vi "PIDcontro2DCmotorUsingMyRio.vi"() -> ()   [LabVIEW 2017]
uses:
  <vilib>/myRIO/Common/Instrument Driver Framework/myRIO v1.0/Encoder/typedefs/Encoder Count Direction Enum.ctl
  <vilib>/myRIO/Common/Instrument Driver Framework/myRIO v1.0/Encoder/typedefs/Encoder Signal Mode.ctl
  <vilib>/myRIO/Instrument Drivers/Onboard IO/Encoder/typedefs/Encoder Reference.ctl
  <vilib>/myRIO/Common/Instrument Driver Framework/Utilities/typedefs/myRIO Generic Hardware Reference.ctl
  <vilib>/myRIO/Common/Instrument Driver Framework/Utilities/typedefs/Hardware Version Enum.ctl
  <vilib>/myRIO/Common/Instrument Driver Framework/Utilities/typedefs/myRIO v1.0 Reference.ctl
  <vilib>/myRIO/Common/Instrument Driver Framework/Utilities/typedefs/Generic FPGA Reference.ctl
  <vilib>/myRIO/Common/Instrument Driver Framework/myRIO v1.0/Encoder/typedefs/Encoder Channels Enum.ctl
  <vilib>/myRIO/Common/Instrument Driver Framework/myRIO v1.0/Encoder/typedefs/Encoder Configuration v1.0.ctl
  <vilib>/userdefined/High Color/nirio_resource_hc.ctl
  <vilib>/myRIO/Instrument Drivers/Onboard IO/PWM/typedefs/PWM Reference.ctl
  <vilib>/myRIO/Common/Instrument Driver Framework/myRIO v1.0/PWM/typedefs/PWM Channels Enum.ctl
  <vilib>/myRIO/Instrument Drivers/Onboard IO/PWM/typedefs/PWM Configuration.ctl
  <vilib>/myRIO/Instrument Drivers/Onboard IO/DIO/typedefs/DIO Reference.ctl
  <vilib>/myRIO/Common/Instrument Driver Framework/myRIO v1.0/DIO/typedefs/DIO Channels List.ctl
  <vilib>/myRIO/Common/Instrument Driver Framework/myRIO v1.0/DIO/typedefs/DIO Channels Enum.ctl
  <vilib>/myRIO/Common/Instrument Driver Framework/Utilities/vis/Is FPGA Ref Available.vi
  <vilib>/myRIO/Common/Instrument Driver Framework/myRIO v1.0/Encoder/vis/myRIO v1.1 Open Encoder.vi
  <vilib>/myRIO/Instrument Drivers/Onboard IO/Encoder/vis/Read.vi
  <vilib>/myRIO/Common/Instrument Driver Framework/myRIO v1.0/PWM/vis/myRIO v1.1 Open PWM.vi
  <vilib>/myRIO/Instrument Drivers/Onboard IO/PWM/vis/Set Duty Cycle and Frequency.vi
  <vilib>/myRIO/Common/Instrument Driver Framework/myRIO v1.0/DIO/vis/myRIO v1.1 Open DIO.vi
  <vilib>/myRIO/Instrument Drivers/Onboard IO/DIO/vis/Write.vi
  <vilib>/myRIO/Common/Instrument Driver Framework/Utilities/vis/Validate Channels.vi
  <vilib>/myRIO/Common/Instrument Driver Framework/myRIO v1.0/Encoder/vis/myRIO v1.0 Reserve Encoder.vi
  <vilib>/myRIO/Common/Instrument Driver Framework/myRIO v1.0/PWM/vis/myRIO v1.0 Reserve PWM.vi
  <vilib>/myRIO/Common/Instrument Driver Framework/myRIO v1.0/DIO/vis/myRIO v1.0 Reserve DIO.vi
  <vilib>/myRIO/Common/Instrument Driver Framework/myRIO v1.0/UART/vis/myRIO v1.0 Close UART.vi
  <vilib>/myRIO/Common/Instrument Driver Framework/myRIO v1.0/Encoder/vis/myRIO v1.0 Build MUX Configuration Encoder.vi
  <vilib>/myRIO/Common/Instrument Driver Framework/myRIO v1.0/Resource Manager/vis/myRIO v1.0 Reserve Channel List.vi
  <vilib>/myRIO/Common/Instrument Driver Framework/myRIO v1.0/PWM/vis/myRIO v1.0 Build MUX Configuration PWM.vi
  <vilib>/myRIO/Common/Instrument Driver Framework/myRIO v1.0/DIO/vis/myRIO v1.0 Build MUX Configuration DIO.vi
  <vilib>/myRIO/Common/Instrument Driver Framework/myRIO v1.0/Resource Manager/vis/myRIO v1.0 Create Configuration List.vi
  <vilib>/myRIO/Common/Instrument Driver Framework/myRIO v1.0/Resource Manager/vis/myRIO v1.0 Reserve Channel.vi
  <vilib>/myRIO/Common/Instrument Driver Framework/myRIO v1.0/Resource Manager/vis/myRIO v1.0 Unreserve Channel.vi
  <vilib>/myRIO/Common/Instrument Driver Framework/myRIO v1.0/Resource Manager/vis/myRIO v1.0 Build Mutex Name.vi
  <vilib>/myRIO/Instrument Drivers/Onboard IO/Encoder/vis/Smart Open.vi
  <vilib>/Utility/error.llb/Error Cluster From Error Code.vi
  <vilib>/myRIO/Common/Instrument Driver Framework/myRIO v1.0/Encoder/vis/myRIO v1.0 Read Encoder.vi
  <vilib>/Utility/VariantDataType/GetNumericInfo.vi
  <vilib>/myRIO/Common/Instrument Driver Framework/myRIO v1.0/myRIO v1.1 Open.vi
  <vilib>/myRIO/Common/Instrument Driver Framework/Utilities/vis/IO Manager.vi
  <vilib>/myRIO/Common/Instrument Driver Framework/Utilities/vis/Configuration Manager.vi
  <vilib>/myRIO/Common/Instrument Driver Framework/myRIO v1.0/Resource Manager/vis/myRIO v1.0 Configure IO.vi
  <vilib>/myRIO/Common/Instrument Driver Framework/myRIO v1.0/myRIO v1.0 Close.vi
  <vilib>/myRIO/Common/Instrument Driver Framework/myRIO v1.0/Encoder/vis/myRIO v1.0 Configure Encoder.vi
  <vilib>/addons/control/pid/pid.llb/PID (DBL).vi
  <vilib>/myRIO/Common/Instrument Driver Framework/myRIO v1.0/PWM/vis/myRIO v1.0 Write PWM.vi
  <vilib>/myRIO/Common/Instrument Driver Framework/myRIO v1.0/DIO/vis/myRIO v1.0 Write DIO.vi
  <vilib>/myRIO/Instrument Drivers/Onboard IO/PWM/vis/Smart Open.vi
  <vilib>/myRIO/Instrument Drivers/Onboard IO/DIO/vis/Smart Open.vi
  <vilib>/myRIO/Common/Instrument Driver Framework/Utilities/vis/FPGA Ref Manager.vi
  <vilib>/myRIO/Common/Instrument Driver Framework/myRIO v1.0/myRIO v1.0 Reset FPGA.vi
  <vilib>/myRIO/Common/Instrument Driver Framework/myRIO v1.0/IRQ/vis/myRIO v1.0 IRQ Info FGV.vi
  <vilib>/myRIO/Common/Instrument Driver Framework/myRIO v1.0/IRQ/vis/myRIO v1.0 Timer IRQ Info FGV.vi
  <vilib>/myRIO/Common/Instrument Driver Framework/myRIO v1.0/IRQ/vis/myRIO v1.0 ISR Agent.vi
  <vilib>/myRIO/Express VI/Onboard IO/Encoder/Encoder Express VI.xnode
  <vilib>/myRIO/Instrument Drivers/Onboard IO/Encoder/vis/myRIO Encoder Open.xnode
  <vilib>/myRIO/Express VI/Onboard IO/PWM/PWM Express VI.xnode
  <vilib>/myRIO/Instrument Drivers/Onboard IO/PWM/vis/myRIO PWM Open.xnode
  <vilib>/myRIO/Express VI/Onboard IO/DO/DO Express VI.xnode
  <vilib>/myRIO/Instrument Drivers/Onboard IO/DIO/vis/myRIO DIO Open.xnode
  <vilib>/myRIO/Instrument Drivers/Utilities/Utilities.lvlib
  <vilib>/addons/control/pid/NI_PID_pid.lvlib
  <vilib>/myRIO/Instrument Drivers/Onboard IO/DIO/DIO.lvlib
  <vilib>/myRIO/Instrument Drivers/Onboard IO/PWM/PWM.lvlib
  <vilib>/myRIO/Instrument Drivers/Onboard IO/Encoder/Encoder.lvlib
panel:
  in  "Enable 2":bool
  out "Direction 2":bool
  out "Counter Value 2":i32
  out "Counter Direction 2":T1
  in  "Reset Counter 2":bool
  out "PPS 2":dbl
  out "RPM 2":dbl
  out "RPS 2":dbl
  out "Motor Response-SetSpeed & ActualSpeed RightM":cluster{"Speed SetPoint":dbl, dbl}(graph)
  out "Motor Right Speed RPM RPM 2":dbl(knob) caption="Gauge" scale=0.0..150.0
  out "Motor Left Speed RPM":dbl(knob) caption="Gauge" scale=0.0..150.0
  out "Motor Response-SetSpeed & ActualSpeed LeftM":cluster{"Speed SetPoint":dbl, dbl}(graph)
  out "RPS":dbl
  out "RPM":dbl
  out "PPS":dbl
  out "Direction":bool
  in  "Enable":bool
  in  "Speed SetPoint":dbl(slide) scale=0.0..106.0
  in  "PWM freq [Hz]":dbl(slide)=100.0 scale=40.0..40000.0
  in  "Reset Counter":bool
  out "Counter Direction":T1
  out "Counter Value":i32
  in  "[ESC]":bool
  # "H-Bridge &  2 Geared Motor demo Real Time control and Tuning using MyRio-1900"
  # "By Abdalrahman M. Amer \nabdalrahman.m5959@Gmail.com"
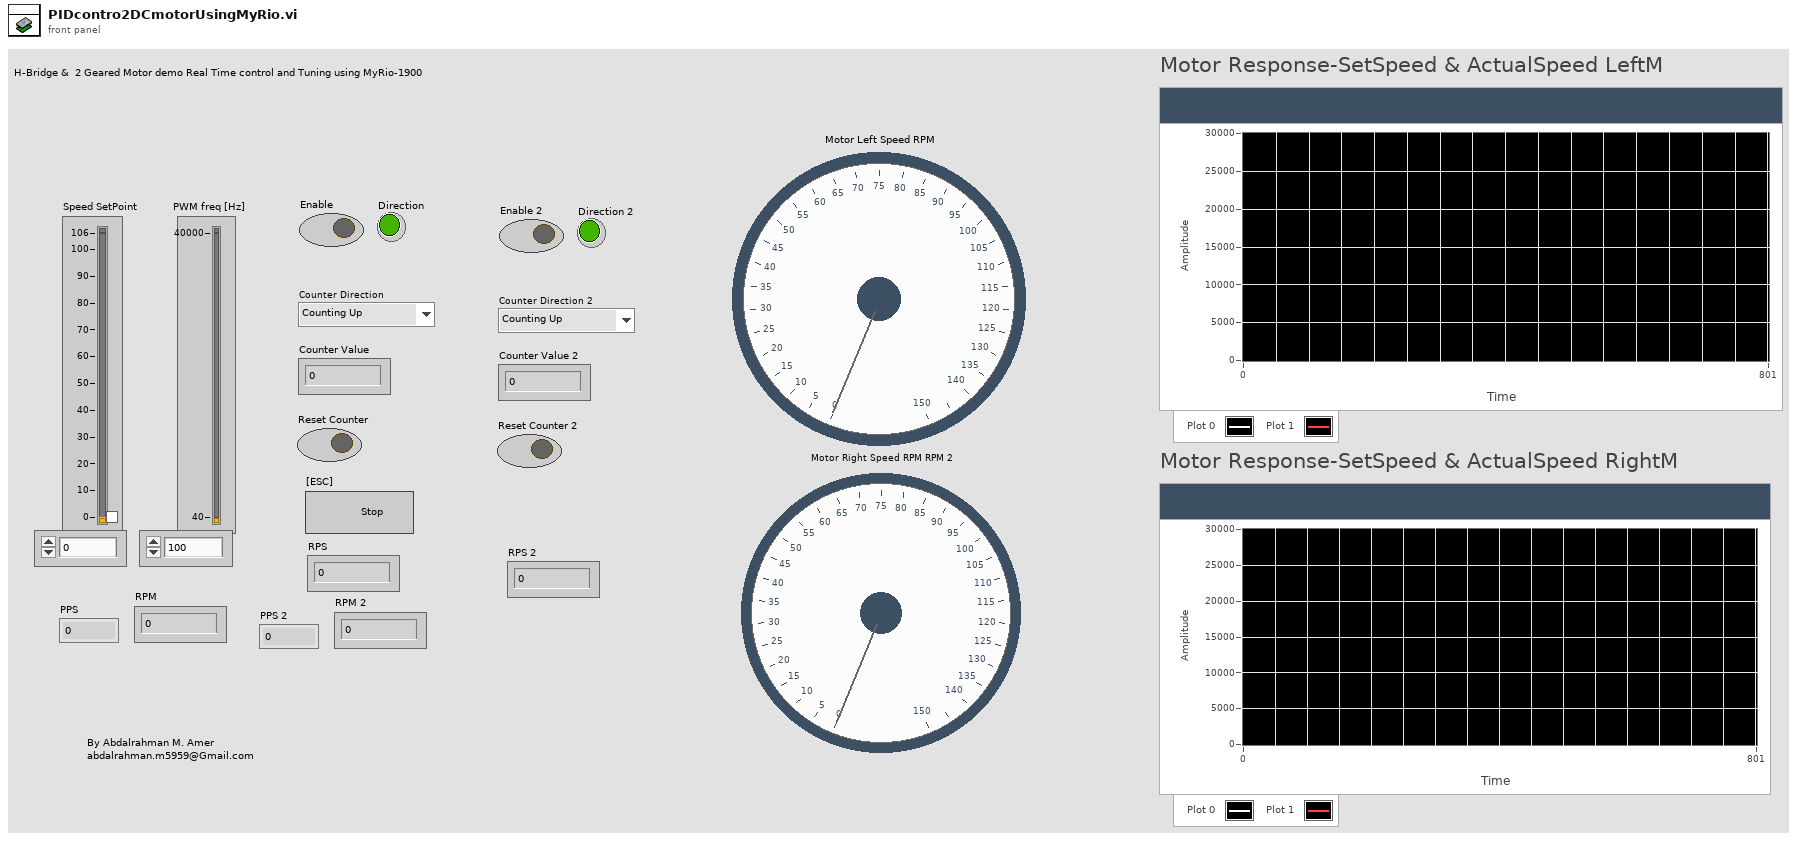
[diagram p1: front panel]
types:
  T1 = typedef "Encoder Count Direction Enum.ctl" = enum16{"Counting Up", "Counting Down"}
  T2 = cluster{"proportional gain (Kc)":dbl, "integral time (Ti, min)":dbl, "derivative time (Td, min)":dbl}
  T3 = typedef "PWM.lvlib/PWM Reference.ctl" = cluster{"myRIO Reference":T4, "PWM Channels Enum":T8, "PWM Configuration":T9}
  T4 = typedef "myRIO Generic Hardware Reference.ctl" = cluster{"myRIO Model":T5, "myRIO Hardware Reference":T6}
  T5 = typedef "Hardware Version Enum.ctl" = enum16{"Unknown", "myRIO-1900", "myRIO-1950", "roboRIO", "NI ELVIS RIO CM"}
  T6 = typedef "myRIO v1.0 Reference.ctl" = cluster{"Generic FPGA Reference":T7, "Allow multiple opens":bool}
  T7 = typedef "Generic FPGA Reference.ctl" = refnum<k20>
  T8 = typedef "PWM Channels Enum.ctl" = enum16{"Not Connected", "C/PWM0", "C/PWM1", "A/PWM0", "A/PWM1", "A/PWM2", "B/PWM0", "B/PWM1", "B/PWM2", "PWM/PWM0", "PWM/PWM1", "PWM/PWM2", "PWM/PWM3", "PWM/PWM4", "PWM/PWM5", "PWM/PWM6", "PWM/PWM7", "PWM/PWM8", "PWM/PWM9"}
  T9 = typedef "PWM.lvlib/PWM Configuration.ctl" = cluster{"Frequency":dbl, "Duty Cycle":dbl}
  T10 = typedef "nirio_resource_hc.ctl" = tag
  T11 = typedef "DIO.lvlib/DIO Reference.ctl" = cluster{"myRIO Reference":T4, "DIO Channels List":T12}
  T12 = typedef "DIO Channels List.ctl" = T13[]
  T13 = typedef "DIO Channels Enum.ctl" = enum16{"Not Connected", "C/DIO0", "C/DIO1", "C/DIO2", "C/DIO3", "C/DIO4", "C/DIO5", "C/DIO6", "C/DIO7", "A/DIO0", "A/DIO1", "A/DIO2", "A/DIO3", "A/DIO4", "A/DIO5", "A/DIO6", "A/DIO7", "A/DIO8", "A/DIO9", "A/DIO10", "A/DIO11", "A/DIO12", "A/DIO13", "A/DIO14", "A/DIO15", "B/DIO0", "B/DIO1", "B/DIO2", "B/DIO3", "B/DIO4", "B/DIO5", "B/DIO6", "B/DIO7", "B/DIO8", "B/DIO9", "B/DIO10", "B/DIO11", "B/DIO12", "B/DIO13", "B/DIO14", "B/DIO15", "LED0", "LED1", "LED2", "LED3", "Button0", "DIO/DIO0", "DIO/DIO1", "DIO/DIO2", "DIO/DIO3", "DIO/DIO4", "DIO/DIO5", "DIO/DIO6", "DIO/DIO7", "DIO/DIO8", "DIO/DIO9", "SPI/CS0", "SPI/CS1", "SPI/CS2", "SPI/CS3", "LED RADIO (Green)", "LED RADIO (Red)", "LED COMM (Green)", "LED COMM (Red)", "LED MODE (Green)", "LED MODE (Red)"}
  T14 = typedef "Encoder.lvlib/Encoder Reference.ctl" = cluster{"myRIO Reference":T4, "Encoder Channels Enum":T15}
  T15 = typedef "Encoder Channels Enum.ctl" = enum16{"Not Connected", "C/ENC0", "C/ENC1", "A/ENC", "B/ENC", "DIO/ENC0", "DIO/ENC1", "DIO/ENC2", "DIO/ENC3", "DIO/ENC4"}
  T16 = typedef "Encoder Signal Mode.ctl" = enum16{"Quadrature phase signal", "Step and direction signal"}
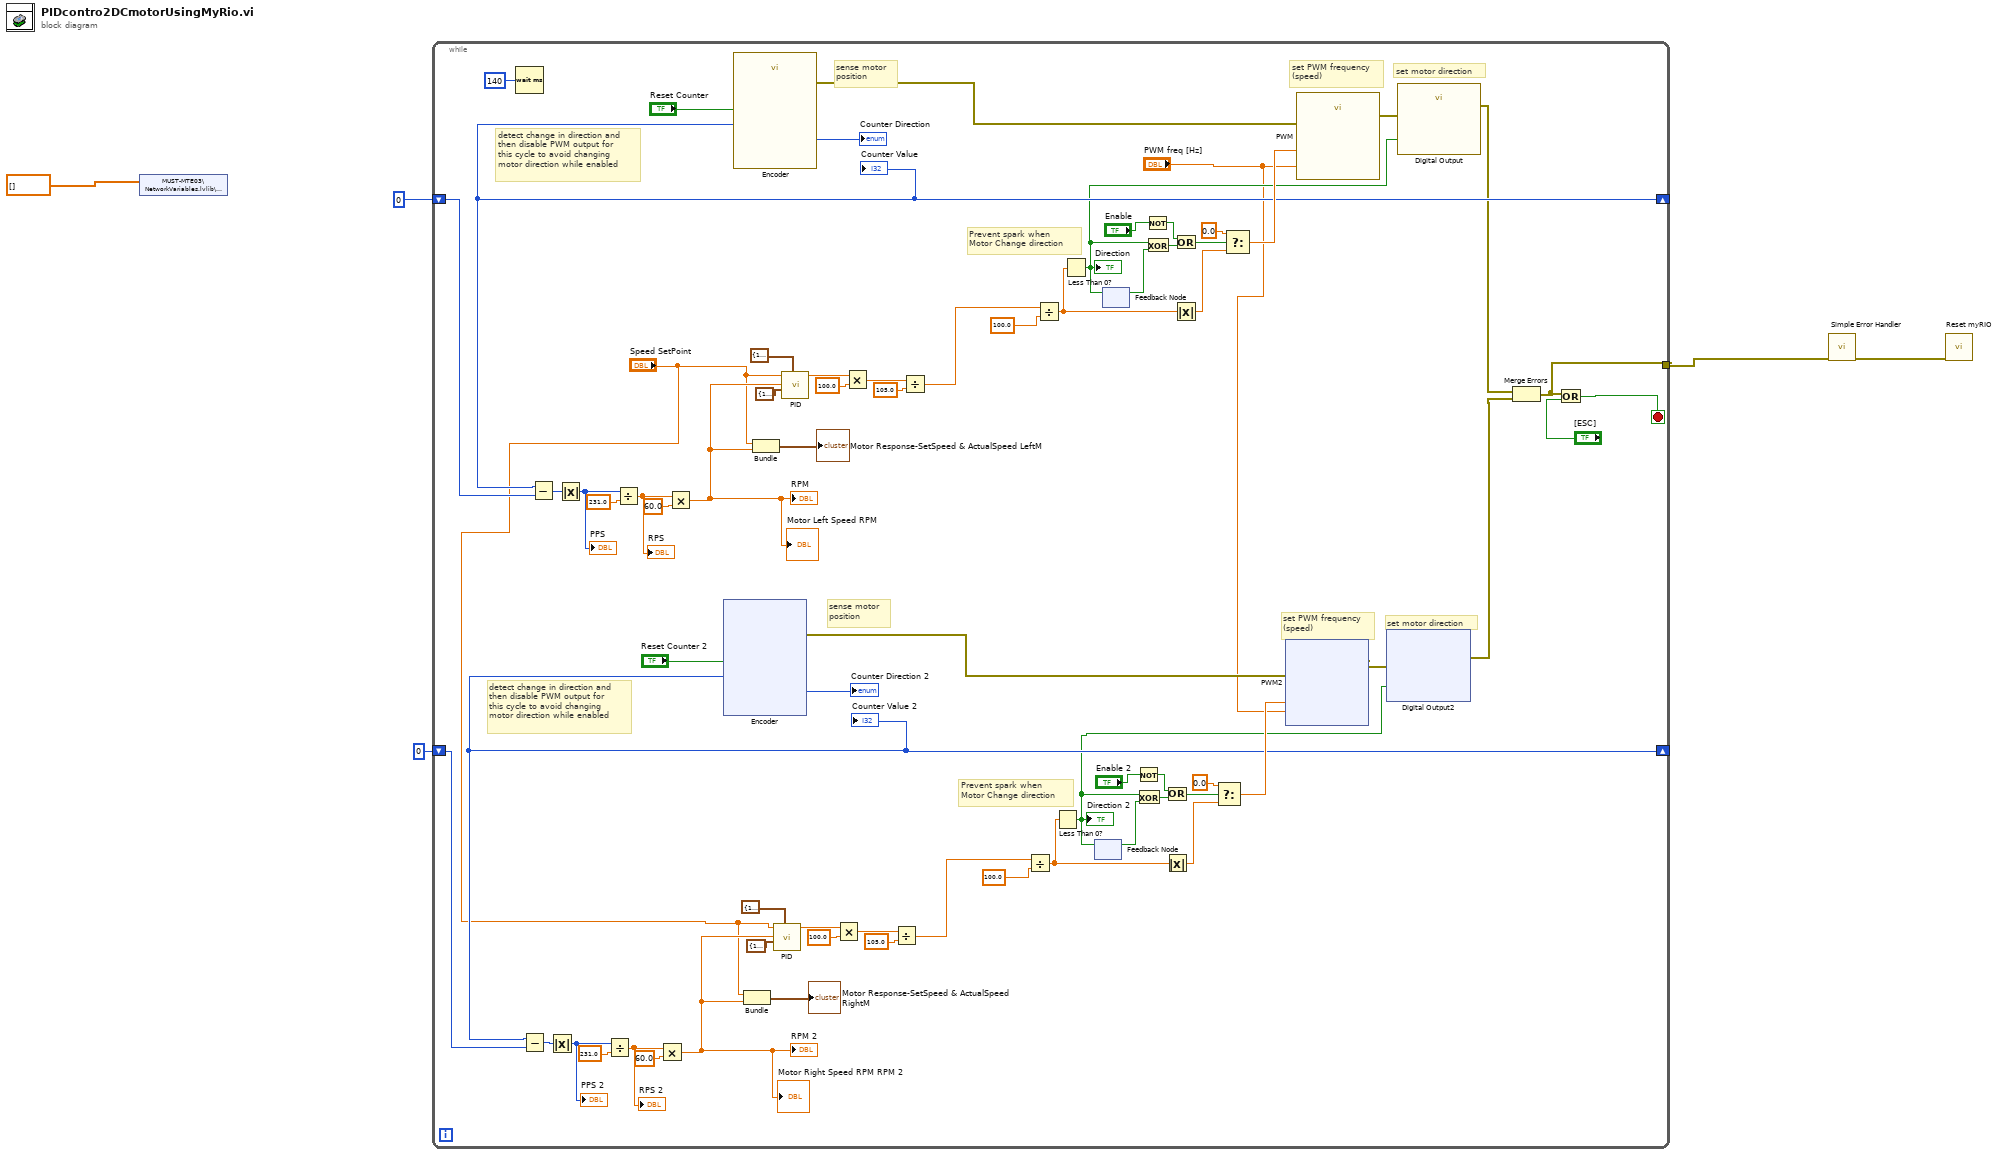
[diagram p0: block diagram]
diagram:
  n1 = shared-variable "MUST-MTE03\\NetworkVariables.lvlib\\RobotPath"(dbl[] [] ("RobotPath")) -> ()  [unwired: 1 in, 1 out]
  n2 = while {
    shift-right: [w53] -> _
    shift-left: 0 ("Counter Value") -> [w54]
    shift-right: [w13] -> _
    shift-left: 0 ("Counter Value") -> [w12]
    tunnel: [w9] -> w1
    stop <- w75 stop-if-true
    # "Prevent spark when \nMotor Change direction"
    # "sense motor \nposition"
    # "detect change in direction and\nthen disable PWM output for\nthis cycle to avoid changing\nmotor direction while enabled"
    # "set PWM frequency\n(speed)"
    # "set motor direction"
    # "Prevent spark when \nMotor Change direction"
    # "sense motor \nposition"
    # "detect change in direction and\nthen disable PWM output for\nthis cycle to avoid changing\nmotor direction while enabled"
    # "set PWM frequency\n(speed)"
    # "set motor direction"
    n3 = Wait (ms)(milliseconds to wait=u32 140) -> ()  [unwired: 1 out]
    n4 = xnode "Encoder"("Reset Counter"="Reset Counter 2") -> ("Counter Value"=w13:i32, "Counter Direction"=→"Counter Direction 2":T1, "error out"=w15:errorcluster)  [unwired: 1 in, 1 out]
    "Counter Value 2" <- w13
    n5 = Subtract(x=w13, y=w12) -> (x-y=w32:i32)
    n6 = Absolute Value(x=w32) -> (abs(x)=w28:i32)
    "PPS 2" <- w28
    n7 = Divide(x=w28, y=231.0) -> (x/y=w31:dbl)
    "RPS 2" <- w31
    n8 = Multiply(x=w31, y=60.0) -> (x*y=w41:dbl)
    "RPM 2" <- w41
    "Motor Right Speed RPM RPM 2" <- w41
    n9 = call "Encoder"("Reset Counter"="Reset Counter") -> ("Counter Value"=w53:i32, "Counter Direction"=→"Counter Direction":T1, "error out"=w72:errorcluster)  [unwired: 23 in, 1 out]
    "Counter Value" <- w53
    n10 = Subtract(x=w53, y=w54) -> (x-y=w52:i32)
    n11 = Absolute Value(x=w52) -> (abs(x)=w58:i32)
    "PPS" <- w58
    n12 = Divide(x=w58, y=231.0) -> (x/y=w55:dbl)
    "RPS" <- w55
    n13 = Multiply(x=w55, y=60.0) -> (x*y=w42:dbl)
    "RPM" <- w42
    "Motor Left Speed RPM" <- w42
    n14 = Bundle("Speed SetPoint"="Speed SetPoint", w41) -> (→"Motor Response-SetSpeed & ActualSpeed RightM":cluster{"Speed SetPoint":dbl, dbl})  [unwired: 1 in]
    n15 = Bundle("Speed SetPoint"="Speed SetPoint", w42) -> (→"Motor Response-SetSpeed & ActualSpeed LeftM":cluster{"Speed SetPoint":dbl, dbl})  [unwired: 1 in]
    n16 = call-poly <vilib>:"PID.vi"("output range"=cluster{"output high":dbl, "output low":dbl} {"output high"=106.0, "output low"=0.0}, "PID gains"=T2 {"proportional gain (Kc)"=1.0, "integral time (Ti, min)"=0.01, "derivative time (Td, min)"=0.0}, "process variable"=w41, "setpoint"="Speed SetPoint") -> ("output"=w34:dbl)  [unwired: 6 in, 1 out]
    n17 = call-poly <vilib>:"PID.vi"("output range"=cluster{"output high":dbl, "output low":dbl} {"output high"=106.0, "output low"=0.0}, "PID gains"=T2 {"proportional gain (Kc)"=1.0, "integral time (Ti, min)"=0.01, "derivative time (Td, min)"=0.0}, "process variable"=w42, "setpoint"="Speed SetPoint") -> ("output"=w50:dbl)  [unwired: 6 in, 1 out]
    n18 = Multiply(x=w34, y=100.0) -> (x*y=w33:dbl)
    n19 = Multiply(x=w50, y=100.0) -> (x*y=w51:dbl)
    n20 = Divide(x=w33, y=105.0) -> (x/y=w40:dbl)
    n21 = Divide(x=w51, y=105.0) -> (x/y=w43:dbl)
    n22 = Divide(x=w40, y=100.0) -> (x/y=w25:dbl)
    n23 = Divide(x=w43, y=100.0) -> (x/y=w62:dbl)
    n24 = Less Than 0?(x=w25) -> (x < 0?=w8:bool)
    "Direction 2" <- w8
    n25 = Less Than 0?(x=w62) -> (x < 0?=w44:bool)
    "Direction" <- w44
    n26 = feedback #1() -> (w17:bool)  [unwired: 1 in]
    n27 = feedback-in #1(w8) -> ()
    n28 = feedback-in #2(w44) -> ()
    n29 = feedback #2() -> (w70:bool)  [unwired: 1 in]
    n30 = Not(x="Enable 2") -> (.not. x?=w22:bool)
    n31 = Exclusive Or(1:w17, 2:w8) -> (0:w19:bool)
    n32 = Not(x="Enable") -> (.not. x?=w65:bool)
    n33 = Exclusive Or(1:w70, 2:w44) -> (0:w68:bool)
    n34 = Or(x=w22, y=w19) -> (x .or. y?=w20:bool)
    n35 = Absolute Value(x=w25) -> (abs(x)=w27:dbl)
    n36 = Or(x=w65, y=w68) -> (x .or. y?=w67:bool)
    n37 = Absolute Value(x=w62) -> (abs(x)=w60:dbl)
    n38 = Select(t=0.0 ("f"), s=w20, f=w27) -> (s? t:f=w26:dbl)
    n39 = Select(t=0.0 ("f"), s=w67, f=w60) -> (s? t:f=w61:dbl)
    n40 = xnode "PWM2"("Duty Cycle"=w26, "Frequency [Hz]"="PWM freq [Hz]", "error in (no error)"=w15) -> ("error out"=w16:errorcluster)
    n41 = call "PWM"("Duty Cycle"=w61, "Frequency [Hz]"="PWM freq [Hz]", "error in (no error)"=w72) -> ("error out"=w71:errorcluster)  [unwired: 24 in]
    n42 = xnode "Digital Output2"("B/DIO0 (Pin 11)"=w8, "error in (no error)"=w16) -> ("error out"=w11:errorcluster)
    n43 = call "Digital Output"("A/DIO0 (Pin 11)"=w44, "error in (no error)"=w71) -> ("error out"=w10:errorcluster)  [unwired: 25 in]
    n44 = Merge Errors(w10, w11) -> (w9:errorcluster)
    n45 = Or(x=w9, y="[ESC]") -> (x .or. y?=w75:bool)
  }
  n46 = call <vilib>:"Simple Error Handler.vi"("error in (no error)"=w1) -> ("error out"=w4:errorcluster)  [unwired: 4 in, 4 out]
  n47 = call <vilib>:"Reset myRIO.vi"("error in (no error)"=w4) -> ()  [unwired: 10 in, 1 out]
